vi "setEventId.vi"(8 "error in (no error)":errorcluster, 10 "eventId":dbl, 11 "ScriptEvent in":refnum<class "ScriptEvent.lvclass">) -> (0 "error out":errorcluster, 3 "ScriptEvent out":refnum<class "ScriptEvent.lvclass">)   [LabVIEW 2009, in "Tools.lvlib" / "Scripting.lvlib" / "ScriptEvent.lvclass"]
uses:
  ScriptEvent.lvclass
  ScriptEvent.lvclass/ScriptEvent.ctl
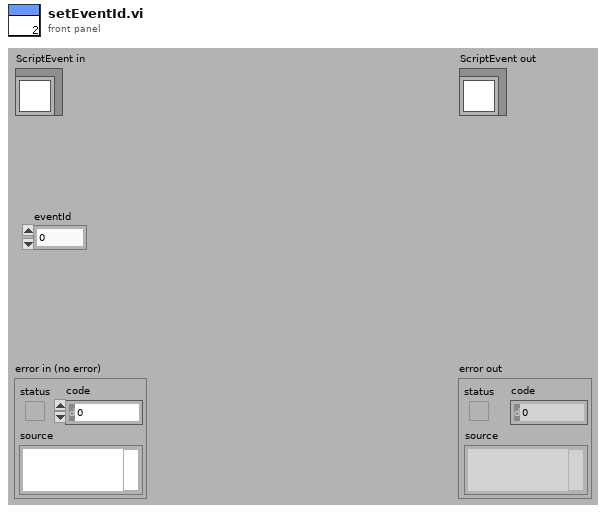
[diagram p1: front panel]
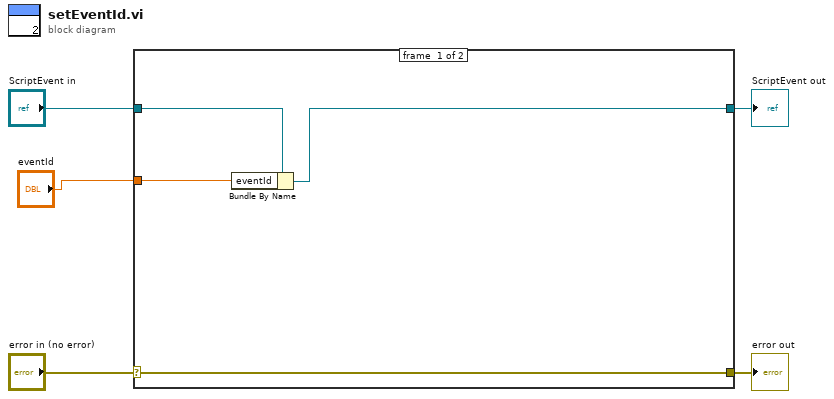
[diagram p0: block diagram]
diagram:
  n1 = case shown="No Error" "error in (no error)" {
    selector: "error in (no error)" -> [w9 w11]
    tunnel: [w9 w11] -> w4
    tunnel: [w7 w10] -> w2
    tunnel: "ScriptEvent in" -> [w8 w10]
    tunnel: "eventId" -> [w6 _]
    frame #0 {
      n2 = Bundle By Name(cluster=w8, "eventId"=w6) -> (w7:refnum<class "ScriptEvent.lvclass">)
    }
    frame #1 {
    }
  }
  "error out" <- w4
  "ScriptEvent out" <- w2
